vi "Beat Sound Octave.vi"() -> ()   [LabVIEW 2021]
doc: "This VI illustrates how to generate and play sine, square, sawtooth and triangle waveforms. You can change the frequency and type of the waveform generated as it plays continuously."
uses:
  <vilib>/sound2/lvsound2.llb/Sampling Mode.ctl
  <vilib>/sound2/lvsound2.llb/Sound Data Format.ctl
  <vilib>/sound2/lvsound2.llb/Sound Output Set Volume (Single).vi
  <vilib>/sound2/lvsound2.llb/Sound Output Write (DBL Single).vi
  <vilib>/measure/NI_MABase.lvlib
panel:
  in  "Frequency 2\n[Hz]":dbl(slide)=0.6000000000000003 min=0.0 max=1000.0 step=0.1 scale=800.0..1000.0
  in  "Frequency 1\n[Hz]":dbl(slide)=0.6000000000000003 min=0.0 max=500.0 step=0.1 scale=430.0..450.0
  in  "Volume":dbl(slide)=21.338912133891213 scale=0.0..100.0
  out "Generated Sound":waveform(dbl)[](graph)=[{"t0"=timestamp(29.931972789115648 s since 1904-01-01), "dt"=2.2675736961451248e-05, "Y"=array[10000 elements], "attributes"=variant("NI_ChannelName"=variant(string "Signal 1"), "NI_ExpIsRelativeTime"=variant(bool TRUE), "NI_ExpStartTimeStamp"=variant(timestamp timestamp(3695136105.7761874 s since 1904-01-01)), "NI_ExpTimeStamp"=variant(timestamp timestamp(3695136135.7081604 s since 1904-01-01)), "NI_ExpXDimension"=variant(string "t"))}, {"t0"=timestamp(29.931972789115648 s since 1904-01-01), "dt"=2.2675736961451248e-05, "Y"=array[10000 elements], "attributes"=variant("NI_ChannelName"=variant(string "Signal 2"), "NI_ExpIsRelativeTime"=variant(bool TRUE), "NI_ExpStartTimeStamp"=variant(timestamp timestamp(3695136105.777132 s since 1904-01-01)), "NI_ExpTimeStamp"=variant(timestamp timestamp(3695136135.709105 s since 1904-01-01)), "NI_ExpXDimension"=variant(string "t"))}, {"t0"=timestamp(29.931972789115648 s since 1904-01-01), "dt"=2.2675736961451248e-05, "Y"=array[10000 elements], "attributes"=variant("NI_ChannelName"=variant(string "Signal 1"), "NI_ExpIsRelativeTime"=variant(bool TRUE), "NI_ExpStartTimeStamp"=variant(timestamp timestamp(3695136105.7761874 s since 1904-01-01)), "NI_ExpTimeStamp"=variant(timestamp timestamp(3695136135.7081604 s since 1904-01-01)), "NI_ExpXDimension"=variant(string "t"))}]
  in  "Stop":bool
  # "Beat Tone Demo"
  # "McClellan et al., DSP First 3-2 Beat Notes"
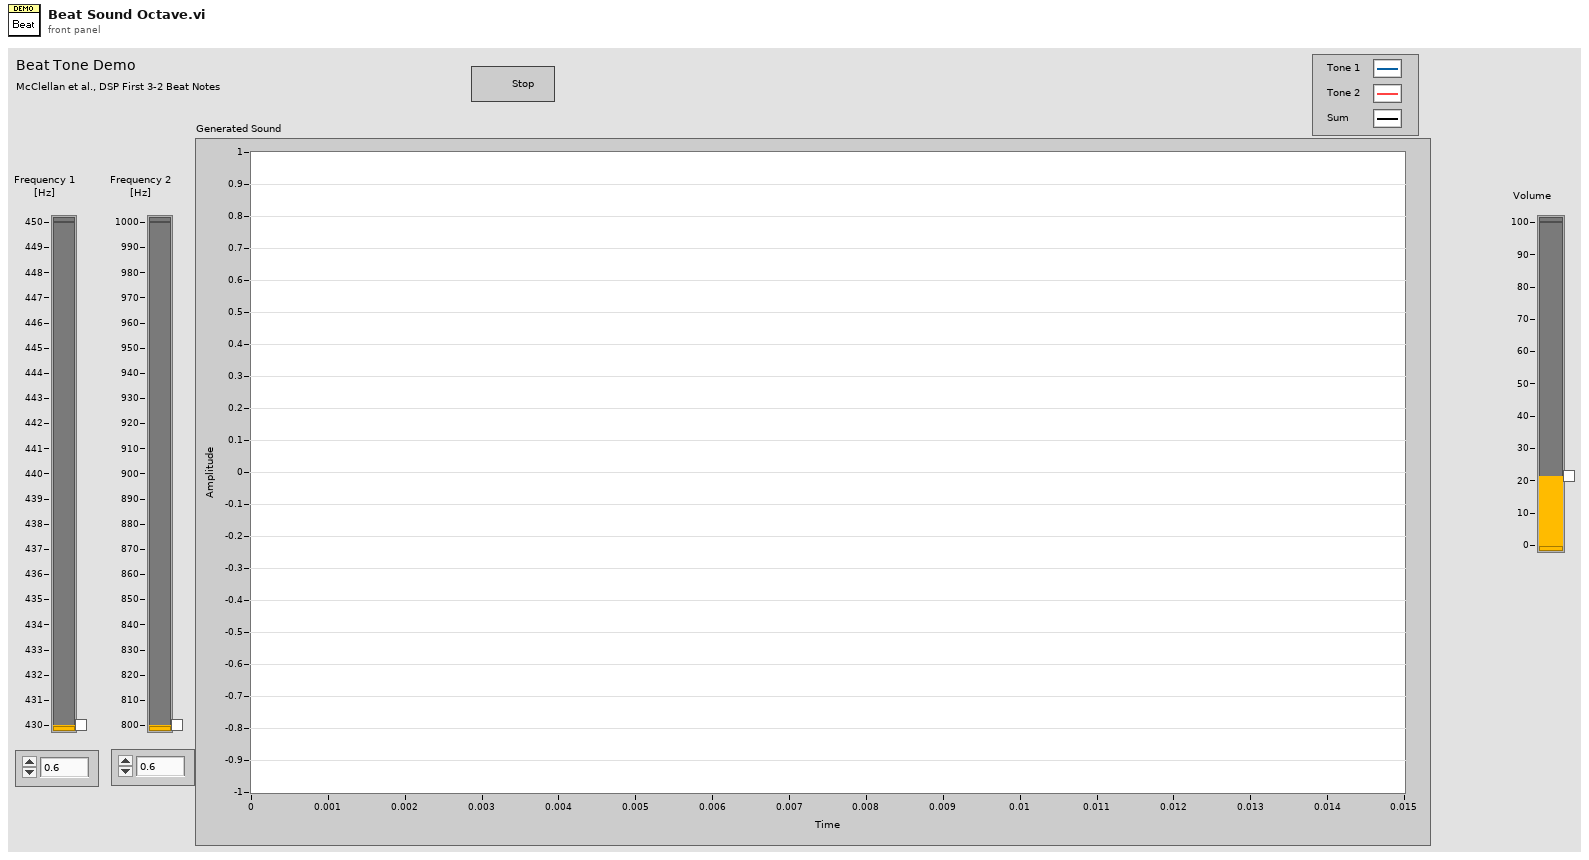
[diagram p1: front panel]
types:
  T1 = typedef "Sound Data Format.ctl" = cluster{"sample rate (S/s)":dbl, "number of channels":i32, "bits per sample":i32}
  T2 = typedef "Sampling Mode.ctl" = i32
  T3 = typedef "Sound Output Task ID.ctl" = u32
  T4 = enum16{"Sine Wave", "Triangle Wave", "Square Wave", "Sawtooth Wave"}
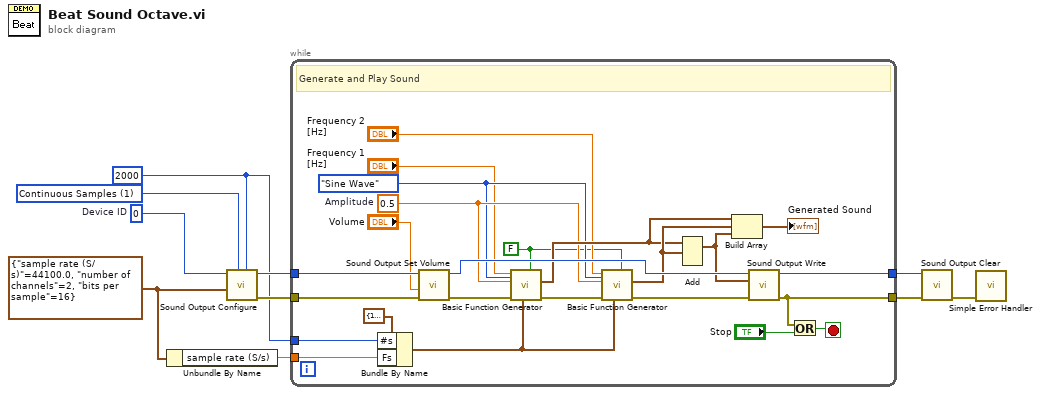
[diagram p0: block diagram]
diagram:
  w6 = u32 0  # Device ID
  w1 = 2000 ("Number of Samples/ch")
  w2 = T1 {"sample rate (S/s)"=44100.0, "number of channels"=2, "bits per sample"=16} ("Sound Format")
  w5 = T2 1 items=["Finite Samples", "Continuous Samples"] ("sample mode")
  n1 = Unbundle By Name(w2) -> ("sample rate (S/s)"=w3:dbl)
  n2 = call <vilib>:"Sound Output Configure.vi"("number of samples/ch"=w1, "sample mode"=w5, "sound format"=w2, "device ID"=w6) -> ("error out"=w10:errorcluster, "task ID"=w9:T3)  [unwired: 6 in]
  n3 = while {
    tunnel: w9 -> [w29]
    tunnel: [w34] -> w7
    tunnel: w10 -> [w31]
    tunnel: [w27] -> w8
    tunnel: w3 -> [w23]
    tunnel: w1 -> [w22]
    stop <- w32 stop-if-true
    w14 = 0.5  # Amplitude
    w12 = FALSE ("reset signal")
    w13 = T4."Sine Wave" ("signal type")
    # "Generate and Play Sound"
    n4 = Bundle By Name(cluster=cluster{"Fs":dbl, "#s":dbl} {"Fs"=1000.0, "#s"=1000.0} ("sampling info"), "#s"=w22, "Fs"=w23) -> (w19:cluster{"Fs":dbl, "#s":dbl})
    n5 = call-poly <vilib>:"Sound Output Set Volume.vi"("error in (no error)"=w31, "volume"="Volume", "task ID"=w29) -> ("error out"=w25:errorcluster, "task ID out"=w30:T3)  [unwired: 7 in]
    n6 = call <vilib>:"Basic Function Generator.vi"("reset signal"=w12, "sampling info"=w19, "signal type"=w13, "error in (no error)"=w25, "amplitude"=w14, "frequency"="Frequency 1\n[Hz]") -> ("error out"=w21:errorcluster, "signal out"=w17:waveform(dbl))  [unwired: 3 in, 1 out]
    n7 = call <vilib>:"Basic Function Generator.vi"("reset signal"=w12, "sampling info"=w19, "signal type"=w13, "error in (no error)"=w21, "amplitude"=w14, "frequency"="Frequency 2\n[Hz]") -> ("error out"=w20:errorcluster, "signal out"=w18:waveform(dbl))  [unwired: 3 in, 1 out]
    n8 = Add(1:w18, 2:w17) -> (0:w16:waveform(dbl))  [unwired: 1 in, 1 out]
    n9 = Build Array(w17, w18, w16) -> (→"Generated Sound":waveform(dbl)[])
    n10 = call-poly <vilib>:"Sound Output Write.vi"("error in (no error)"=w20, "data"=w16, "task ID"=w30) -> ("error out"=w27:errorcluster, "task ID out"=w34:T3)  [unwired: 7 in]
    n11 = Or(x=w27, y="Stop") -> (x .or. y?=w32:bool)
  }
  n12 = call <vilib>:"Sound Output Clear.vi"("error in (no error)"=w8, "task ID"=w7) -> ("error out"=w4:errorcluster)  [unwired: 9 in]
  n13 = call <vilib>:"Simple Error Handler.vi"("error in (no error)"=w4) -> ()  [unwired: 4 in, 5 out]
